vi "Read State.vi"(8 "error in (no error)":errorcluster, 11 "A Context State in":refnum<class "A Context State.lvclass">) -> (0 "error out":errorcluster, 2 "State":refnum<class "State Pattern.lvclass">, 3 "A Context State out":refnum<class "A Context State.lvclass">)   [LabVIEW 2021, in "Context Actor.lvlib" / "A Context State.lvclass"]
uses:
  A Context State.lvclass
  State Pattern/State Pattern.lvclass
  A Context State.lvclass/A Context State.ctl
  Context Actor.lvclass
  C:/PPLs/Design-Patterns/State Pattern/State Pattern/State Pattern.lvclass
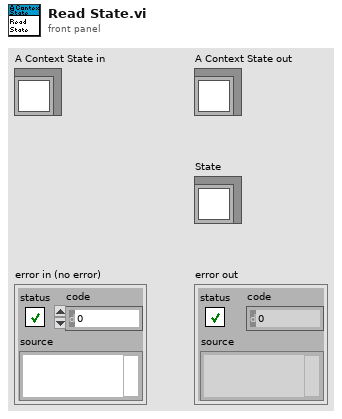
[diagram p1: front panel]
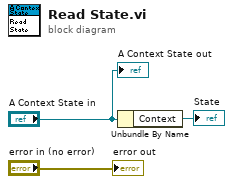
[diagram p0: block diagram]
diagram:
  n1 = Unbundle By Name("A Context State in") -> ("Context"=→"State":refnum<class "Context Actor.lvclass">)
  "error out" <- "error in (no error)"
  "A Context State out" <- "A Context State in"
